vi "Replace_Array_Subset_2D_Element.vi"(9 "Element RAS":i8, 10 "Indexs RAS":T1={"Rows"=-1, "Columns"=-1} {"Columns" min=-1; "Rows" min=-1}, 11 "RAS2D":i8[][](array[numeric])) -> (3 "New Array RAS2D":i8[][](array[numeric]))   [LabVIEW 2018]
uses:
  Controls/Rows_Columns.ctl
panel:
  out "Columns":i32
  out "Rows":i32
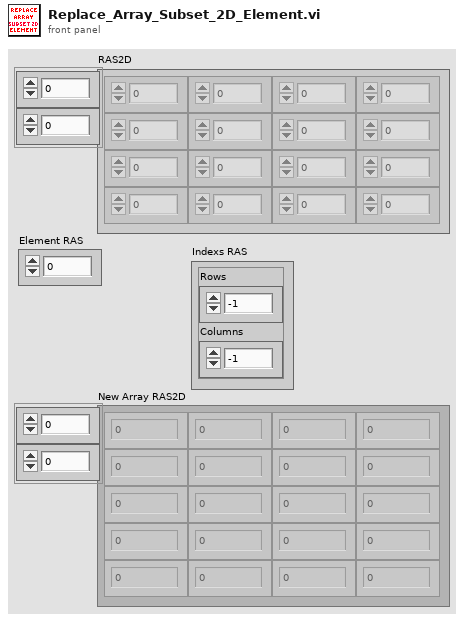
[diagram p1: front panel]
types:
  T1 = typedef "Rows_Columns.ctl" = cluster{"Rows":i32, "Columns":i32}
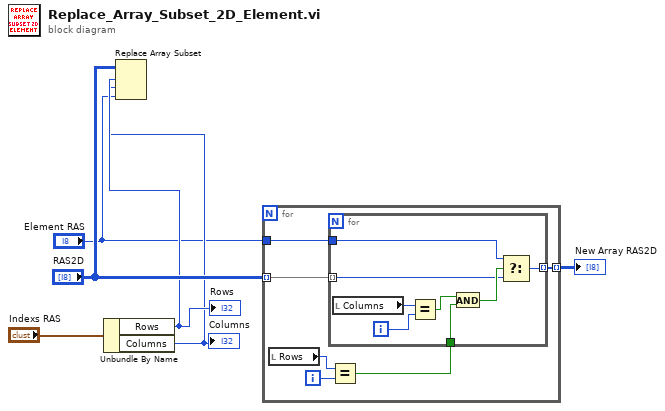
[diagram p0: block diagram]
diagram:
  n1 = Unbundle By Name("Indexs RAS") -> ("Rows"=w4:i32, "Columns"=w3:i32)
  "Rows" <- w4
  "Columns" <- w3
  n2 = Replace Array Subset(array="RAS2D", new element="Element RAS", index (row)=w4, index (col)=w3) -> ()  [unwired: 1 out]
  n3 = for {
    tunnel: "RAS2D" -> [w12] mode=indexing
    tunnel: [w11] -> w2 mode=indexing
    tunnel: "Element RAS" -> [w7]
    i -> [w9]
    n4 = local read "Rows"() -> (w10:i32)
    n5 = Equal?(x=w10, y=w9) -> (x = y?=w8:bool)
    n6 = for {
      tunnel: w12 -> [w14] mode=indexing
      tunnel: [w20] -> w11 mode=indexing
      tunnel: w8 -> [w15]
      tunnel: w7 -> [w13]
      i -> [w16]
      n7 = local read "Columns"() -> (w17:i32)
      n8 = Equal?(x=w17, y=w16) -> (x = y?=w18:bool)
      n9 = And(x=w18, y=w15) -> (x .and. y?=w19:bool)
      n10 = Select(t=w13, s=w19, f=w14) -> (s? t:f=w20:i8)
    }
  }
  "New Array RAS2D" <- w2
